vi "UDP - Receiver.vi"(6 "Maximum Iterations (-1=Inf)":i32=-1, 11 "Receiver Port":u16=50001) -> (3 "Numerics (DBL)":dbl[](array[numeric]) format="%#_10f")   [LabVIEW 2020, in "Data Sharing Framework Scripting Examples.lvlib"]
doc: "The UDP protocol differs from TCP in that there is no error-checking with the packets of information that are sent, and thus no guarantee whatsoever that an intended recipient will actually receive a given piece of data.\n\nThis UDP Receiver VI connects to a port and reads and converts datagrams sent by VeriStand when running the system definition created by Import Data Sharing Framework with UDP Component VI."
uses:
  Data Sharing Framework Scripting Examples.lvlib
panel:
  out "Unsigned Byte Array":u8[][](array[numeric])
  out "Received String Data":string
  in  "Stop":bool
  # "Overview: Demonstrates the use of the UDP functions to receive data over a UDP connection.\nInstructions:\n1. Run the Import Data Sharing Framework with UDP Component example VI to configure a VeriStand system definition to send data to destination port 50001. From VeriStand, deploy the system definition file to start sharing data.\n2. Configure Receiver Port to match destination port (50001).\n2. Run this VI to connect to the specified receiver port using the UDP API and then convert data to the expected format."
  # "Van"
  # "Vbn"
  # "Vcn"
  # "Ia"
  # "Ib"
  # "Ic"
  # "In"
  # "Vdc"
  # "Idc"
  # "count"
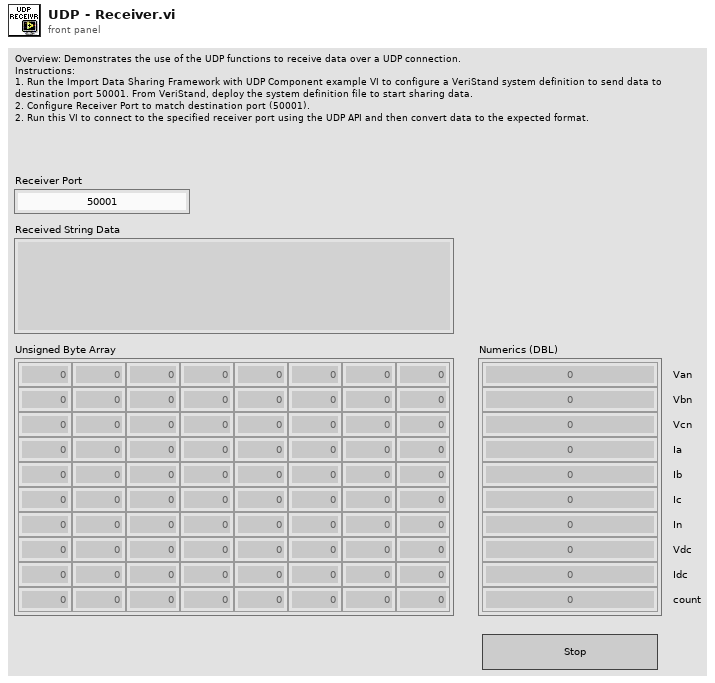
[diagram p1: front panel]
types:
  T1 = enum16{"big-endian, network order", "native, host order", "little-endian"}
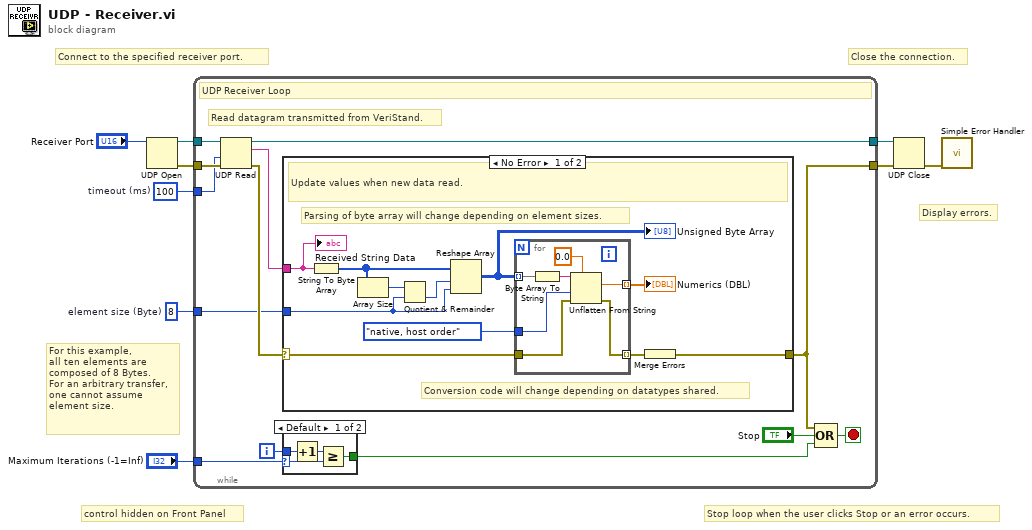
[diagram p0: block diagram]
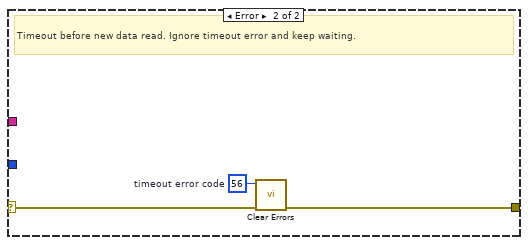
[diagram p3: hidden frame]
diagram:
  w2 = 8  # element size (Byte)
  w3 = 100  # timeout (ms)
  # "control hidden on Front Panel"
  # "For this example,\nall ten elements are \ncomposed of 8 Bytes. \nFor an arbitrary transfer, \none cannot assume \nelement size."
  # "Display errors."
  # "Stop loop when the user clicks Stop or an error occurs."
  # "Close the connection."
  # "Connect to the specified receiver port."
  n1 = UDP Open(11:"Receiver Port") -> (port=w5:refnum<k16>, 0:w6:errorcluster)  [unwired: 4 in, 1 out]
  n2 = while {
    tunnel: w5 -> [w22]
    tunnel: [w15] -> w9
    tunnel: w6 -> [w19]
    tunnel: [w16] -> w7
    tunnel: w3 -> [w14]
    tunnel: w2 -> [w13]
    tunnel: "Maximum Iterations (-1=Inf)" -> [w10]
    i -> [w12]
    stop <- w20 stop-if-true
    # "Read datagram transmitted from VeriStand."
    # "UDP Receiver Loop"
    n3 = UDP Read(connection ID=w22, timeout ms (25000)=w14, 8:w19) -> (data out=w18:string, error out=w17:errorcluster, 3:w15:refnum<k16>)  [unwired: 3 out]
    n4 = case shown="No Error" w17 {
      selector: w17 -> [w27 w46]
      tunnel: w18 -> [w37 _]
      tunnel: [w31 w45] -> w16
      tunnel: w13 -> [w33 _]
      frame No Error {
        # "Parsing of byte array will change depending on element sizes."
        # "Conversion code will change depending on datatypes shared."
        # "Update values when new data read."
        n5 = String To Byte Array(string=w37) -> (unsigned byte array=w35:u8[])
        n6 = Array Size(array=w35) -> (size(s)=w36:i32)
        n7 = Quotient & Remainder(x=w36, y=w33) -> (floor(x/y)=w34:i32)  [unwired: 1 out]
        n8 = Reshape Array(w35, w34, w33) -> (w30:u8[][])
        "Unsigned Byte Array" <- w30
        n9 = for {
          tunnel: w30 -> [w44] mode=indexing
          tunnel: [w42] -> w29 mode=indexing
          tunnel: w27 -> [w40]
          tunnel: [w39] -> w32 mode=indexing
          tunnel: T1."native, host order" ("byte order (0:big-endian, network order)") -> [w38]
          n10 = Byte Array To String(unsigned byte array=w44) -> (string=w43:string)
          n11 = Unflatten From String(type=0.0, binary string=w43, byte order (0:big-endian, network order)=w38, error in (no error)=w40) -> (value=w42:dbl, error out=w39:errorcluster)  [unwired: 1 in, 1 out]
        }
        "Numerics (DBL)" <- w29
        n12 = Merge Errors(w32) -> (w31:errorcluster)
        "Received String Data" <- w37
      }
      frame Error {
        w47 = 56  # timeout error code
        # "Timeout before new data read. Ignore timeout error and keep waiting."
        n13 = call <vilib>:"Clear Errors.vi"("error in (no error)"=w46, "specific error code to clear (0: all)"=w47) -> ("error out"=w45:errorcluster)  [unwired: 4 in, 1 out]
      }
    }
    n14 = case shown="Default" w10 {
      selector: w10 -> [w25 _]
      tunnel: w12 -> [w26 _]
      tunnel: [w24 _] -> w11
      frame Default {
        n15 = Increment(x=w26) -> (x+1=w23:i32)
        n16 = Greater Or Equal?(x=w23, y=w25) -> (x >= y?=w24:bool)
      }
      frame ..-1 {
      }
    }
    n17 = Compound Arithmetic op=OR(w16, "Stop", w11) -> (w20:bool)
  }
  n18 = UDP Close(connection ID=w9, 8:w7) -> (error out=w8:errorcluster)  [unwired: 1 out]
  n19 = call <vilib>:"Simple Error Handler.vi"("error in (no error)"=w8) -> ()  [unwired: 1 in, 8 out]
